vi "Simulator.vi"() -> ()   [LabVIEW 2014]
panel:
  out "Channel Array Out":T1(array[cluster])
  out "Iteration":i32
  out "Ratio":dbl[](array[numeric])
  out "Channel Error":errorcluster
  out "Receiver Error":errorcluster
  out "element":T2
  out "Source Error":errorcluster
  in  "stop":bool
  in  "Channel Array":T1(array[cluster])=[{"Bandwidth(bps)"=1200, "Propagation Delay(ms)"=2, "ChannelQueue"=refnum, "Average Arrival(bps)"=0.0}, {"Bandwidth(bps)"=5000, "Propagation Delay(ms)"=3, "ChannelQueue"=refnum, "Average Arrival(bps)"=0.0}, {"Bandwidth(bps)"=20000, "Propagation Delay(ms)"=10, "ChannelQueue"=refnum, "Average Arrival(bps)"=0.0}, {"Bandwidth(bps)"=1000, "Propagation Delay(ms)"=0, "ChannelQueue"=refnum, "Average Arrival(bps)"=0.0}] {"Bandwidth(bps)" format="%.1p"}
  in  "Tab Control":enum32{"Source", "Splitter"}(tab)
  in  "Path Number":i32=4
  in  "file path":path=path "I:/05.0旅/非线性优化/Project/Simulation/abc.txt"
  in  "method":enum16{"FileInput", "Direct"}(ring)
  in  "AverageSize(bytes)":i32=200
  in  "SizeJitter(bytes)":i32=50
  in  "Time Duration(ms)":u32(slide)=200 scale=0.0..500.0
  out "Packet Number":i32
  out "Remained\nData":u8[](array[numeric])
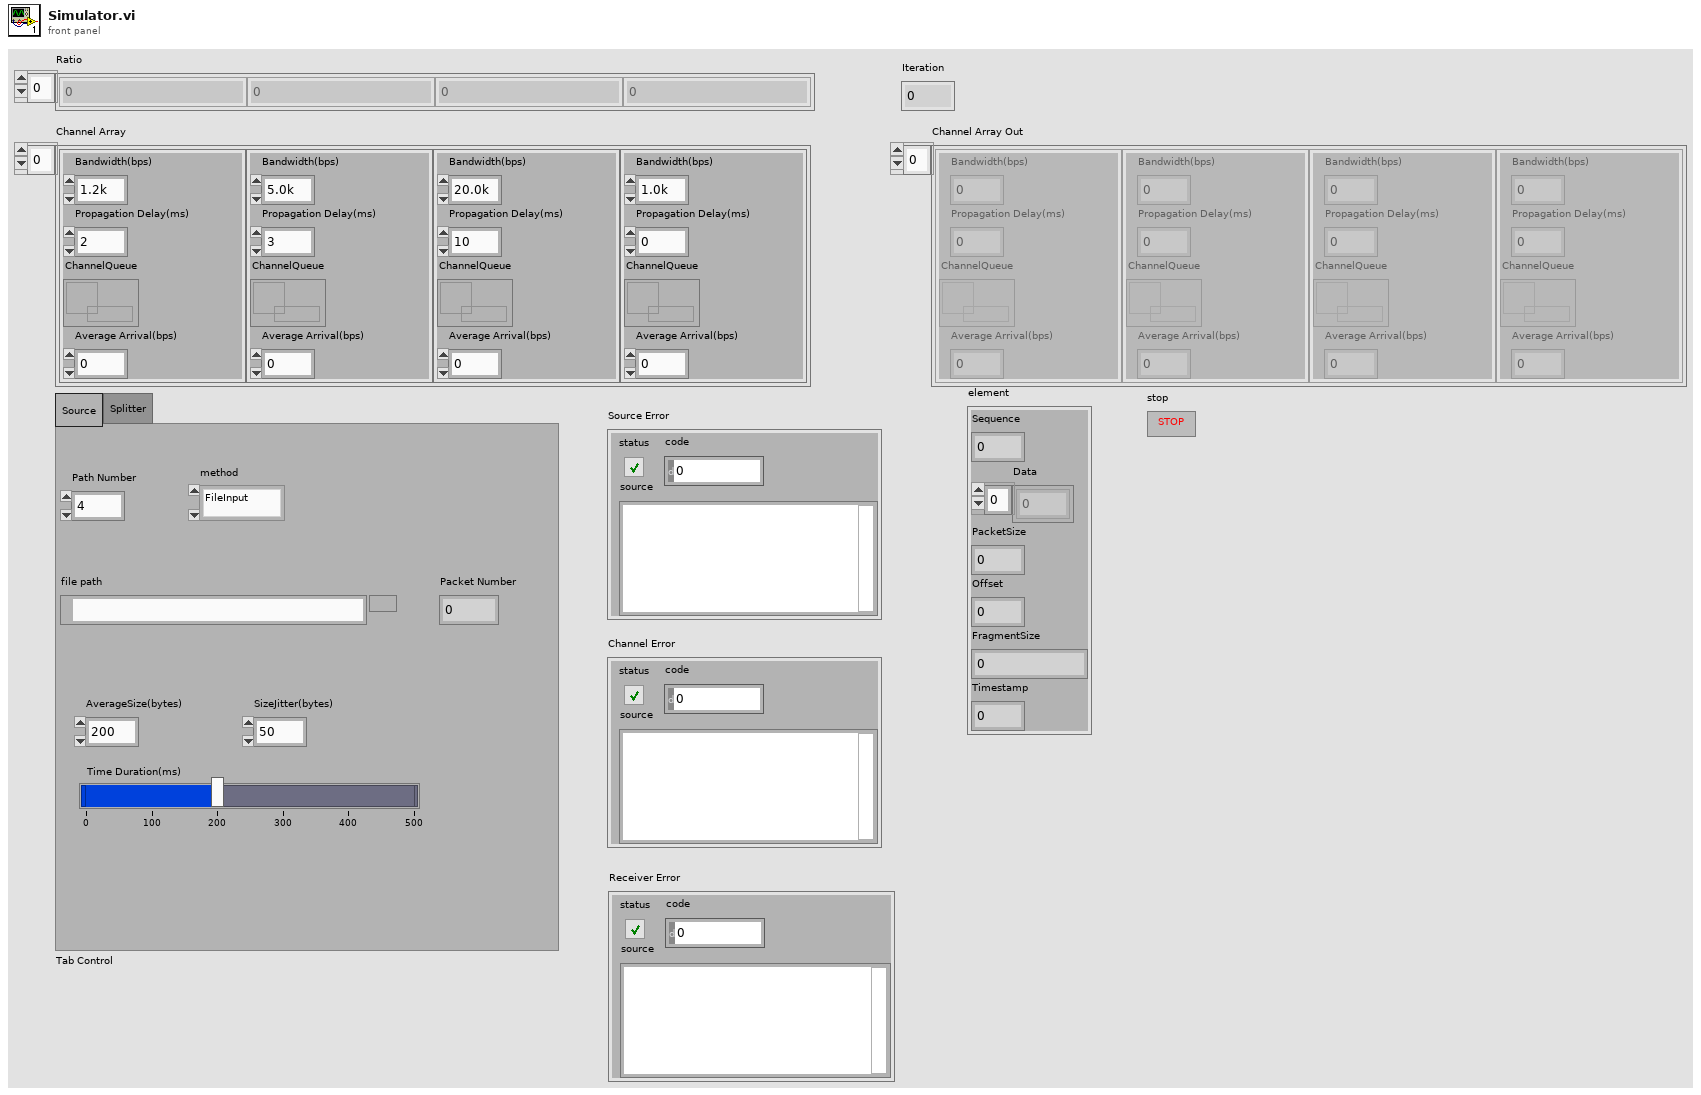
[diagram p1: front panel]
types:
  T1 = cluster{"Bandwidth(bps)":i32, "Propagation Delay(ms)":i32, "ChannelQueue":refnum<queue>, "Average Arrival(bps)":dbl}[]
  T2 = cluster{"Sequence":i32, "Data":u8[], "PacketSize":i32, "Offset":i32, "FragmentSize":i32, "Timestamp":i32}
  T3 = cluster{"Sequence":i32, "Data":u8[], "Timestamp":i32}
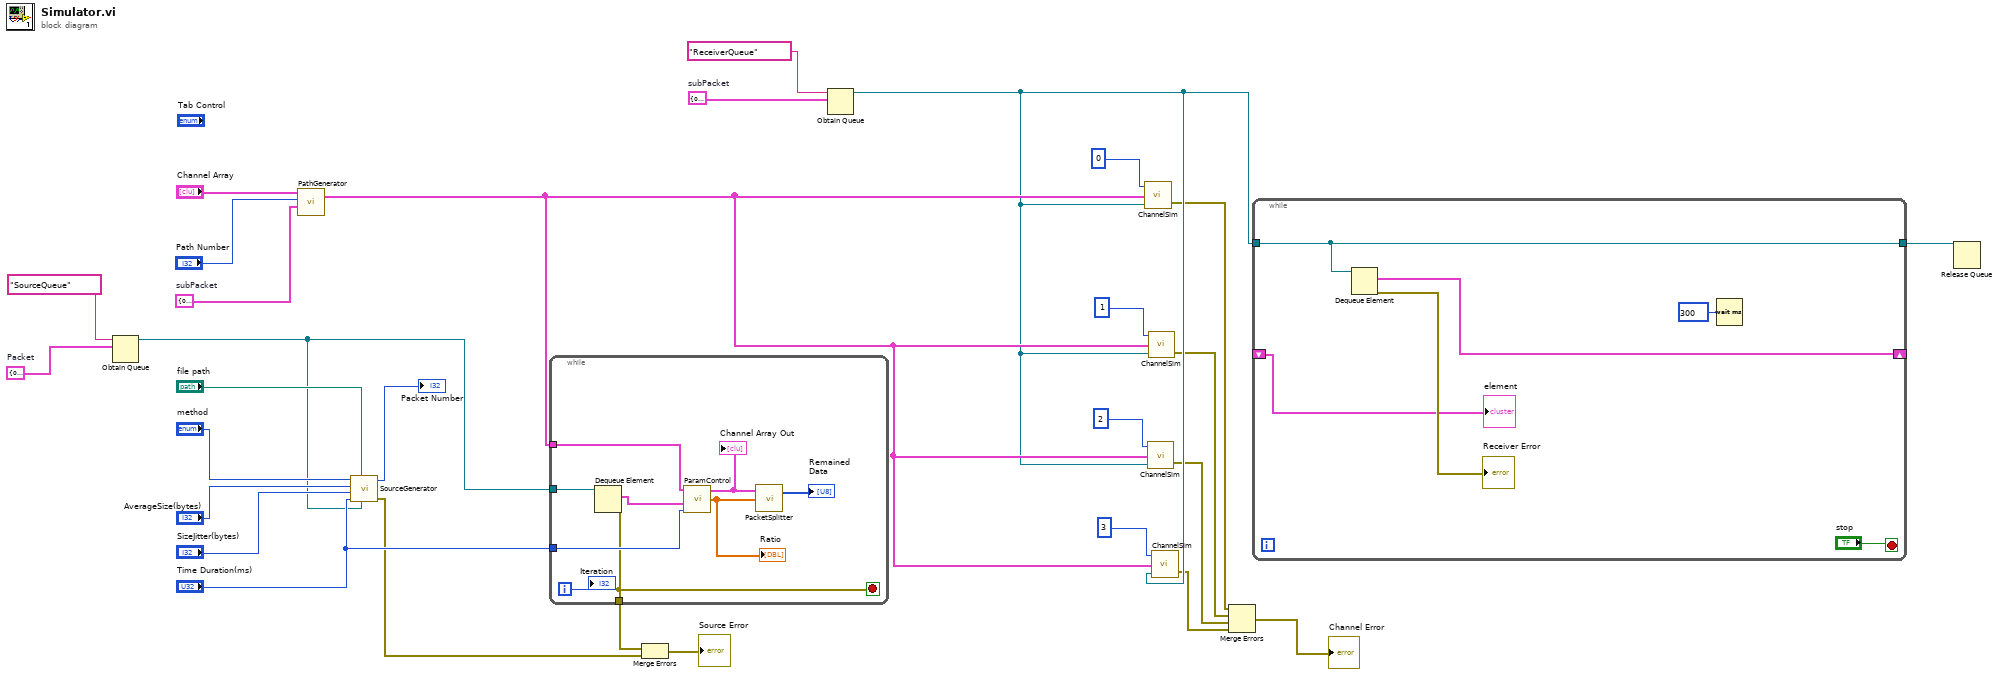
[diagram p0: block diagram]
diagram:
  w5 = T3 {"Sequence"=0, "Data"=[], "Timestamp"=0}  # Packet
  w16 = T2 {"Sequence"=0, "Data"=[], "PacketSize"=0, "Offset"=0, "FragmentSize"=0, "Timestamp"=0}  # subPacket
  w24 = T2 {"Sequence"=0, "Data"=[], "PacketSize"=0, "Offset"=0, "FragmentSize"=0, "Timestamp"=0}  # subPacket
  n1 = Obtain Queue(name (unnamed)="SourceQueue", element data type=w5) -> (queue out=w4:refnum<queue>)  [unwired: 3 in, 2 out]
  n2 = call "PathGenerator.vi"("data type"=w24, "number"="Path Number", "Channel Array In"="Channel Array") -> ("Channel Array Out"=w18:T1)  [unwired: 1 in, 1 out]
  n3 = call "SourceGenerator.vi"("method"="method", "file path"="file path", "AverageSize(bytes)"="AverageSize(bytes)", "SizeJitter(bytes)"="SizeJitter(bytes)", "SourceQueue"=w4, "Time Duration(ms)"="Time Duration(ms)") -> ("size"=→"Packet Number":i32, "error out"=w2:errorcluster)  [unwired: 1 in]
  n4 = while {
    tunnel: w18 -> [w38]
    tunnel: w4 -> [w30]
    tunnel: "Time Duration(ms)" -> [w34]
    tunnel: [w32] -> w3
    i -> [w31]
    stop <- w32 stop-if-true
    n5 = Dequeue Element(queue=w30) -> (element=w33:T3, error out=w32:errorcluster)  [unwired: 2 in, 2 out]
    n6 = call "ParamControl.vi"("Time Duration(ms)"=w34, "Packet"=w33, "Channel Array In"=w38) -> ("Ratio"=w36:dbl[], "Channel Array Out"=w37:T1)  [unwired: 2 in]
    "Ratio" <- w36
    "Channel Array Out" <- w37
    n7 = call "PacketSplitter.vi"("Ratio"=w36, "Channel Array In"=w37) -> ("Remained\nData"=→"Remained\nData":u8[])  [unwired: 2 in]
    "Iteration" <- w31
  }
  n8 = Merge Errors(w3, w2) -> (→"Source Error":errorcluster)
  n9 = Obtain Queue(name (unnamed)="ReceiverQueue", element data type=w16) -> (queue out=w15:refnum<queue>)  [unwired: 3 in, 2 out]
  n10 = call "ChannelSim.vi"("Receiver Queue"=w15, "Channel Array In"=w18, "index"=0) -> ("error out"=w12:errorcluster)  [unwired: 2 in]
  n11 = call "ChannelSim.vi"("Receiver Queue"=w15, "Channel Array In"=w18, "index"=2) -> ("error out"=w10:errorcluster)  [unwired: 2 in]
  n12 = call "ChannelSim.vi"("Receiver Queue"=w15, "Channel Array In"=w18, "index"=1) -> ("error out"=w11:errorcluster)  [unwired: 2 in]
  n13 = call "ChannelSim.vi"("Receiver Queue"=w15, "Channel Array In"=w18, "index"=3) -> ("error out"=w9:errorcluster)  [unwired: 2 in]
  n14 = Merge Errors(w12, w11, w10, w9) -> (→"Channel Error":errorcluster)
  n15 = while {
    tunnel: w15 -> [w41]
    tunnel: [w41] -> w13
    shift-right: [w40] -> _
    shift-left: _ -> [w39]
    stop <- "stop" stop-if-true
    n16 = Dequeue Element(queue=w41) -> (element=w40:T2, error out=→"Receiver Error":errorcluster)  [unwired: 2 in, 2 out]
    n17 = Wait (ms)(milliseconds to wait=u32 300) -> ()  [unwired: 1 out]
    "element" <- w39
  }
  n18 = Release Queue(queue=w13) -> ()  [unwired: 2 in, 3 out]
